vi "Config Curve Point.vi"(0 "VISA resource name":refnum<visa-resource-name>, 1 "Units Value (0.0000)":dbl min=-9999.9999 max=9999.9999 step=0.0001 format="%.4f", 5 "Curve (21)":dbl=21.0 min=21.0 max=28.0 step=1.0, 7 "Index (1)":dbl=1.0 min=1.0 max=200.0 step=1.0, 9 "Temperature Value (0.0000)":dbl min=-9999.9999 max=9999.9999 step=0.0001 format="%.4f", 11 "error in (no error)":errorcluster) -> (4 "VISA resource name out":refnum<visa-resource-name>, 15 "error out":errorcluster)   [LabVIEW 2017, in "Lake Shore Cryotronics 218.lvlib"]
doc: "This VI Configures a user curve point."
uses:
  Lake Shore Cryotronics 218.lvlib
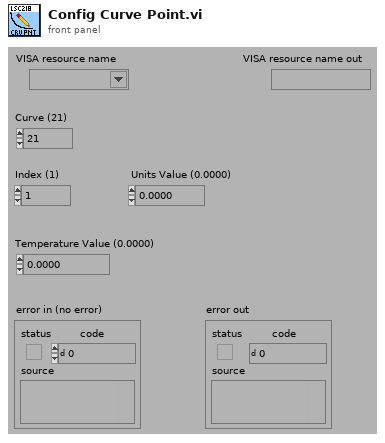
[diagram p1: front panel]
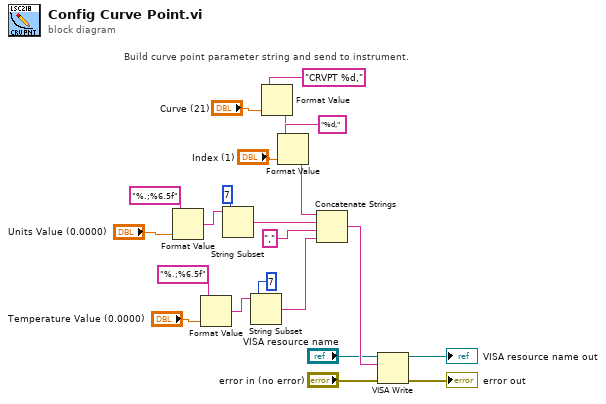
[diagram p0: block diagram]
diagram:
  # "Build curve point parameter string and send to instrument."
  n1 = Format Value(format string="%.;%6.5f", value (0)="Units Value (0.0000)") -> (output string=w16:string)  [unwired: 1 in]
  n2 = Format Value(format string="%.;%6.5f", value (0)="Temperature Value (0.0000)") -> (output string=w9:string)  [unwired: 1 in]
  n3 = String Subset(string=w16, length (rest)=7) -> (substring=w12:string)  [unwired: 1 in]
  n4 = String Subset(string=w9, length (rest)=7) -> (substring=w6:string)  [unwired: 1 in]
  n5 = Format Value(format string="CRVPT %d,", value (0)="Curve (21)") -> (output string=w19:string)  [unwired: 1 in]
  n6 = Format Value(string ("")=w19, format string="%d,", value (0)="Index (1)") -> (output string=w13:string)
  n7 = Concatenate Strings(w13, w12, ",", w6) -> (w5:string)
  n8 = VISA Write(VISA resource name="VISA resource name", write buffer=w5, error in (no error)="error in (no error)") -> (VISA resource name out=→"VISA resource name out":refnum<visa-resource-name>, error out=→"error out":errorcluster)  [unwired: 1 out]
